vi "Read Power Setpoint.vi"   [LabVIEW 2023, in "Power Control.lvclass"]
uses:
  Power Control.lvclass
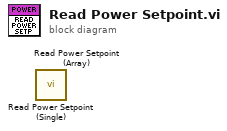
[diagram p0: block diagram]
diagram:
  n1 = call "Read Power Setpoint (Single).vi"() -> ()  [unwired: 8 in, 4 out]
  n2 = call "Read Power Setpoint (Array).vi"() -> ()  [unwired: 8 in, 4 out]
